vi "FP_monitor.vi"() -> ()   [LabVIEW 2017]
panel:
  in  "选项卡控件":enum32{"PT status", "Alarm Params"}(tab)
  out "OVL?":bool[](array[boolean])
  out "PT values":dbl[](array[numeric])
  out "realtime error msg":string
  out "last emailed msg":string
  out "emailed num":u32
  in  "update interval (s)":i32=5 min=5
  in  "Leidon IP address":string="127.0.0.1"
  out "Version of exe":string
  in  "停止":bool
  in  "Mute?":bool
  in  "Alarm params":T1(array[cluster])=[{"min"=0.5, "max"=1.5, "normal msg"="PT is ON (good)", "overlevel msg"="PT is OFF !!!"}, {"min"=0.0, "max"=40.0, "normal msg"="water out is cool (good)", "overlevel msg"="water out is too hot !!!"}]
  # "ON(1)/OFF(0)"
  # "T water out (C)"
  # "outrange -> beep\nstatus changed -> email & mute off\nemail address -> FP_monitor_config.ini"
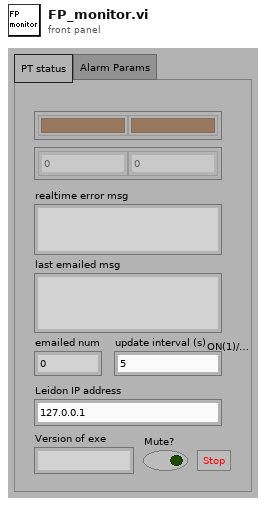
[diagram p1: front panel]
types:
  T1 = cluster{"min":dbl, "max":dbl, "normal msg":string, "overlevel msg":string}[]
  T2 = cluster{"host":string, "port":i32, "username":string, "password":string, "From":string, "to":string, "subject":string}
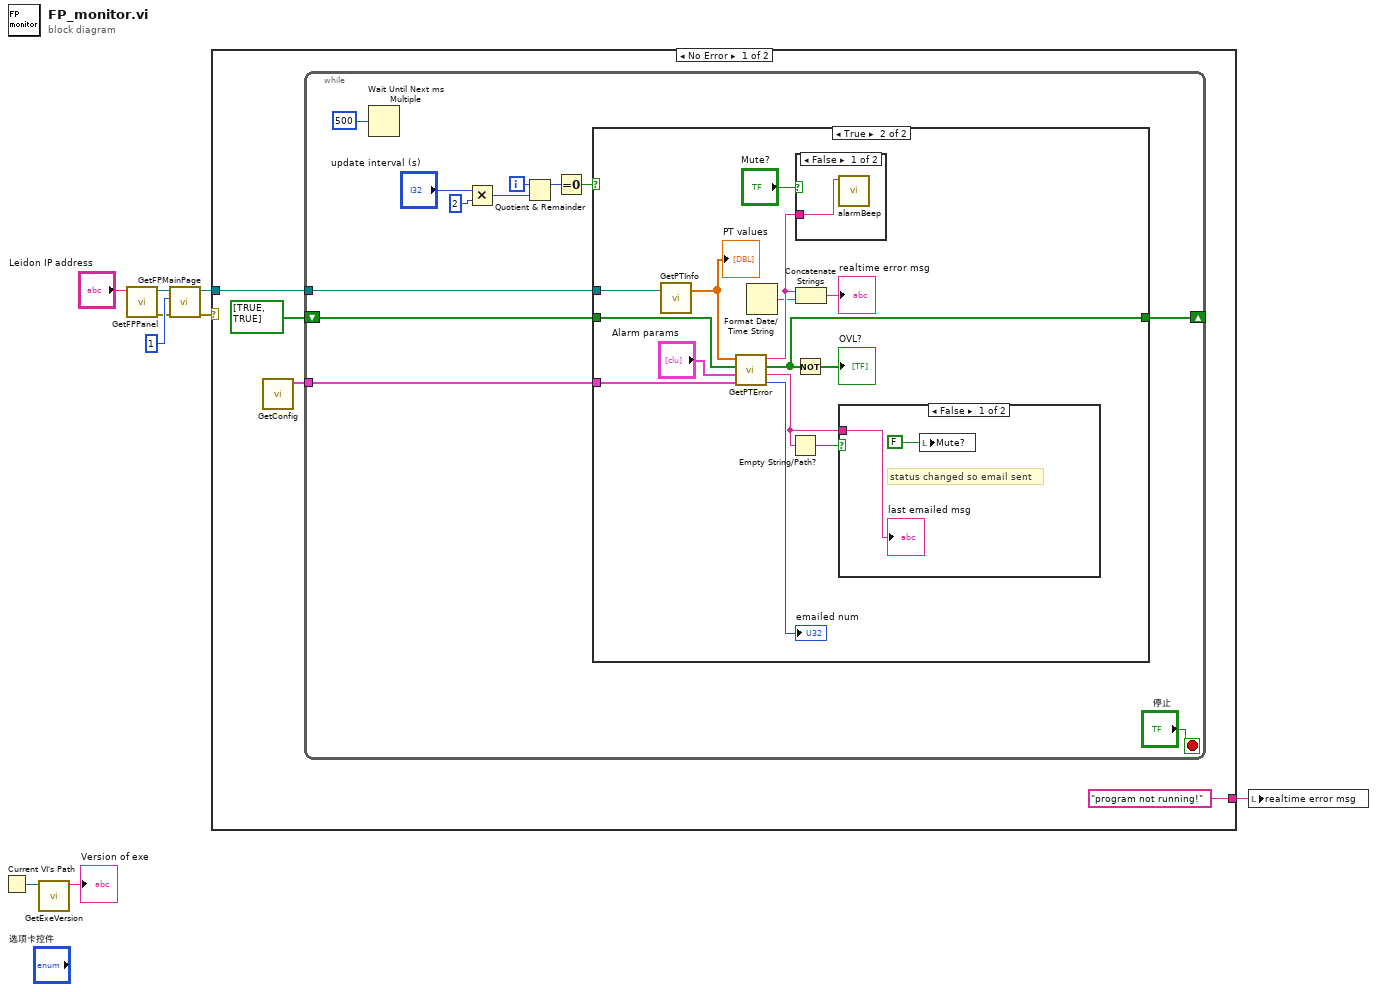
[diagram p0: block diagram]
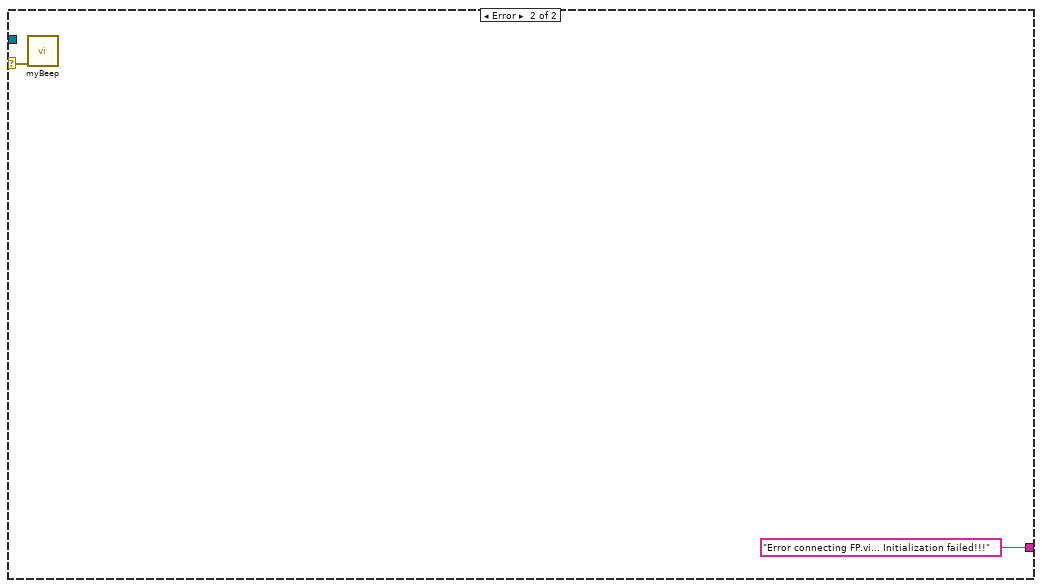
[diagram p5: hidden frame]
diagram:
  n1 = Current VI's Path() -> (path=w3:path)
  n2 = call "GetExeVersion.vi"("路径"=w3) -> ("Version of Executable"=→"Version of exe":string)  [unwired: 10 out]
  n3 = call "GetFPPanel.vi"("机器名(\"\": 打开本地引用)"="Leidon IP address") -> ("错误输出"=w7:errorcluster, "Panel"=w8:refnum<vi>)  [unwired: 1 in, 6 out]
  n4 = call "GetFPMainPage.vi"("错误输入（无错误）"=w7, "索引"=1, "Panel"=w8) -> ("错误输出"=w5:errorcluster, "Page引用句柄"=w6:refnum<vi>)  [unwired: 5 out]
  n5 = case shown="No Error" w5 {
    selector: w5 -> [_ w45]
    tunnel: w6 -> [w13 _]
    tunnel: ["program not running!" ("error msg") "Error connecting FP.vi... Initialization failed!!!" ("error string")] -> w1
    frame No Error {
      n6 = call "GetConfig.vi"() -> ("mail info out"=w10:T2)  [unwired: 11 out]
      n7 = while {
        tunnel: w13 -> [w24]
        shift-right: [w16] -> _
        shift-left: bool[] [TRUE, TRUE] ("errors out (new)") -> [w15]
        tunnel: w10 -> [w14]
        i -> [w23]
        stop <- "停止" stop-if-true
        n8 = Wait Until Next ms Multiple(millisecond multiple=u32 500 ("毫秒倍数")) -> ()  [unwired: 1 out]
        n9 = Multiply(x="update interval (s)", y=2) -> (x*y=w18:i32)
        n10 = Quotient & Remainder(x=w23, y=w18) -> (x-y*floor(x/y)=w22:i32)  [unwired: 1 out]
        n11 = Equal To 0?(x=w22) -> (x = 0?=w21:bool)
        n12 = case shown="True" w21 {
          tunnel: w24 -> [_ w40]
          tunnel: [w26 w30] -> w16
          tunnel: w15 -> [w26 w39]
          tunnel: w14 -> [_ w28]
          frame False {
          }
          frame True {
            n13 = call "GetPTInfo.vi"("Page引用句柄"=w40) -> ("PT values"=w33:dbl[])  [unwired: 1 in, 1 out]
            "PT values" <- w33
            n14 = call "GetPTError.vi"("mail info"=w28, "params"="Alarm params", "normal? (in, old)"=w39, "PT values"=w33) -> ("emailed number"=→"emailed num":u32, "last emailed msg"=w38:string, "normal? (out, new)"=w30:bool[], "overlevel msg"=w36:string)  [unwired: 2 out]
            n15 = Format Date/Time String() -> (date/time string=w35:string)  [unwired: 3 out]
            n16 = Empty String/Path?(string/path=w38) -> (empty?=w37:bool)
            n17 = Not(x=w30) -> (.not. x?=→"OVL?":bool[])
            n18 = case shown="False" "Mute?" {
              tunnel: w36 -> [w41 _]
              frame False {
                n19 = call "alarmBeep.vi"("Error msg"=w41) -> ()  [unwired: 11 out]
              }
              frame True {
              }
            }
            n20 = Concatenate Strings(w36, w35) -> (→"realtime error msg":string)
            n21 = case shown="False" w37 {
              tunnel: w38 -> [w43 _]
              frame False {
                # "status changed so email sent"
                n22 = local write "Mute?"(FALSE ("Mute?")) -> ()
                "last emailed msg" <- w43
              }
              frame True {
              }
            }
          }
        }
      }
    }
    frame Error {
      n23 = call "myBeep.vi"("error in (no error)"=w45) -> ()  [unwired: 11 out]
    }
  }
  n24 = local write "realtime error msg"(w1) -> ()
